vi "VendingMachine.vi"() -> ()   [LabVIEW 2022 SP3]
uses:
  <vilib>/Utility/error.llb/DialogType.ctl
  <vilib>/Instr/_visa.llb/VISA Configure Serial Port (Instr).vi
  Globalne_zmienne.vi
panel:
  out "UstalonaCena1 2":dbl=1.4256114757235e-311
  out "UstalonaCena2":dbl
  out "UstalonaCena3 2":dbl
  out "UstalonaCena4":dbl
  out "Cena 12":dbl
  out "Cena 11":dbl
  out "Cena 10":dbl
  out "Cena 9":dbl
  out "Cena 8":dbl
  out "Cena 6":dbl
  out "Cena 4":dbl
  out "Cena 5":dbl
  out "Cena 3":dbl
  out "Cena 2":dbl
  out "Cena":dbl
  out "Cena 7":dbl=1.4256114754706e-311
  in  "Ustronianka":dbl
  in  "Tarczyn":dbl
  in  "Tiger":dbl
  in  "Black":dbl
  in  "Muszynianka":dbl
  in  "Tymbark":dbl
  in  "Cappy":dbl
  in  "Nestea":dbl
  in  "Mountain Dew":dbl
  in  "Kofola":dbl
  in  "Pepsi":dbl
  in  "Coca-Cola":dbl
  out "Symulacja wydania napoju":bool
  out "Wplacone pieniadze":i32
  out "2,5":bool
  out "3":bool
  out "4,5":bool
  out "5":bool
  out "Reszta":dbl
  in  "5zl":bool
  in  "2zl":bool
  in  "1zl":bool
  out "Wybierz Numer:":i32
  in  "VISA in":refnum<visa-resource-name>
  # "Koszt wybranego napoju"
  # "Proponowane:\nUstalona cena1 = 5\nUstalona cena2 =4,5\nUstalona cena3= 3\nUstalona cena4= 2,5"
  # "Instrukcja:\n*Ustaw BoundRate na mikrokontrolerze na 228800\n\n*Ustal cene i VISA port po lewej stronie\n*Ustaw numery produktow na unikatowe dla kazdej pozycji\n\n*Za pomoca przyciskow S2 i S3 wybierz \nodpowiedni produkt\n\n*Za pomoca przyciskow wplac pieniadze\n\n*Zatwierz podwójnie przyciskajac S4"
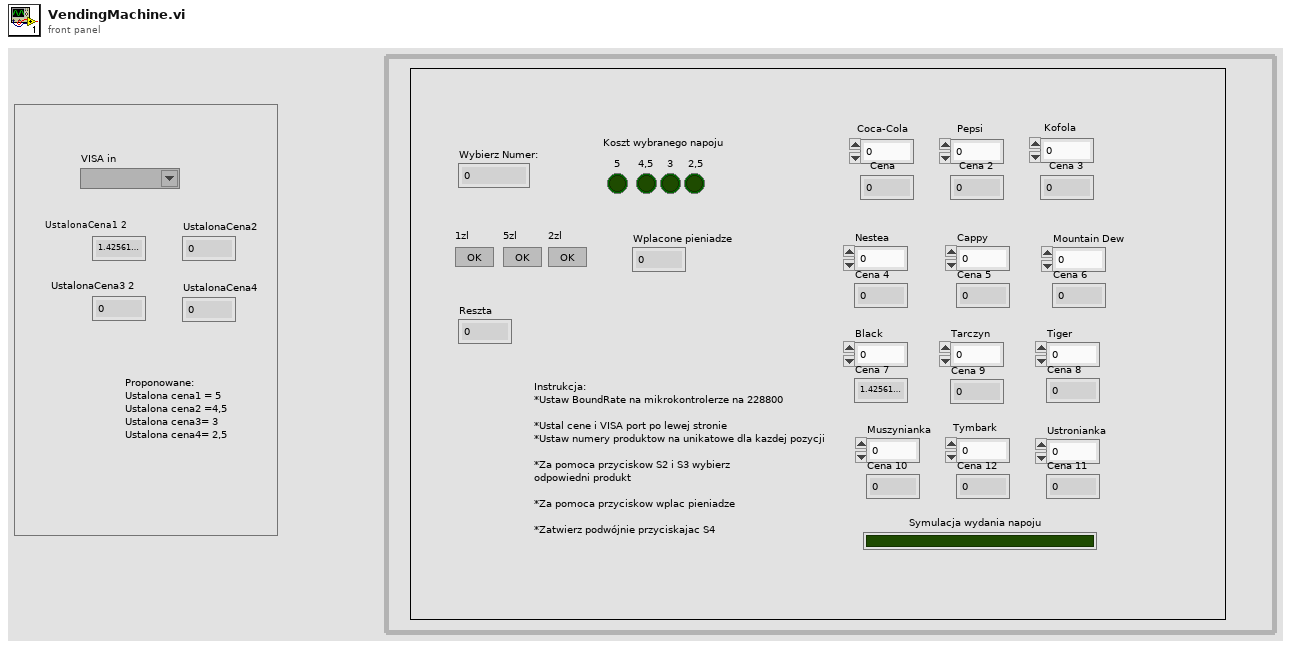
[diagram p1: front panel]
types:
  T1 = typedef "DialogType.ctl" = u16
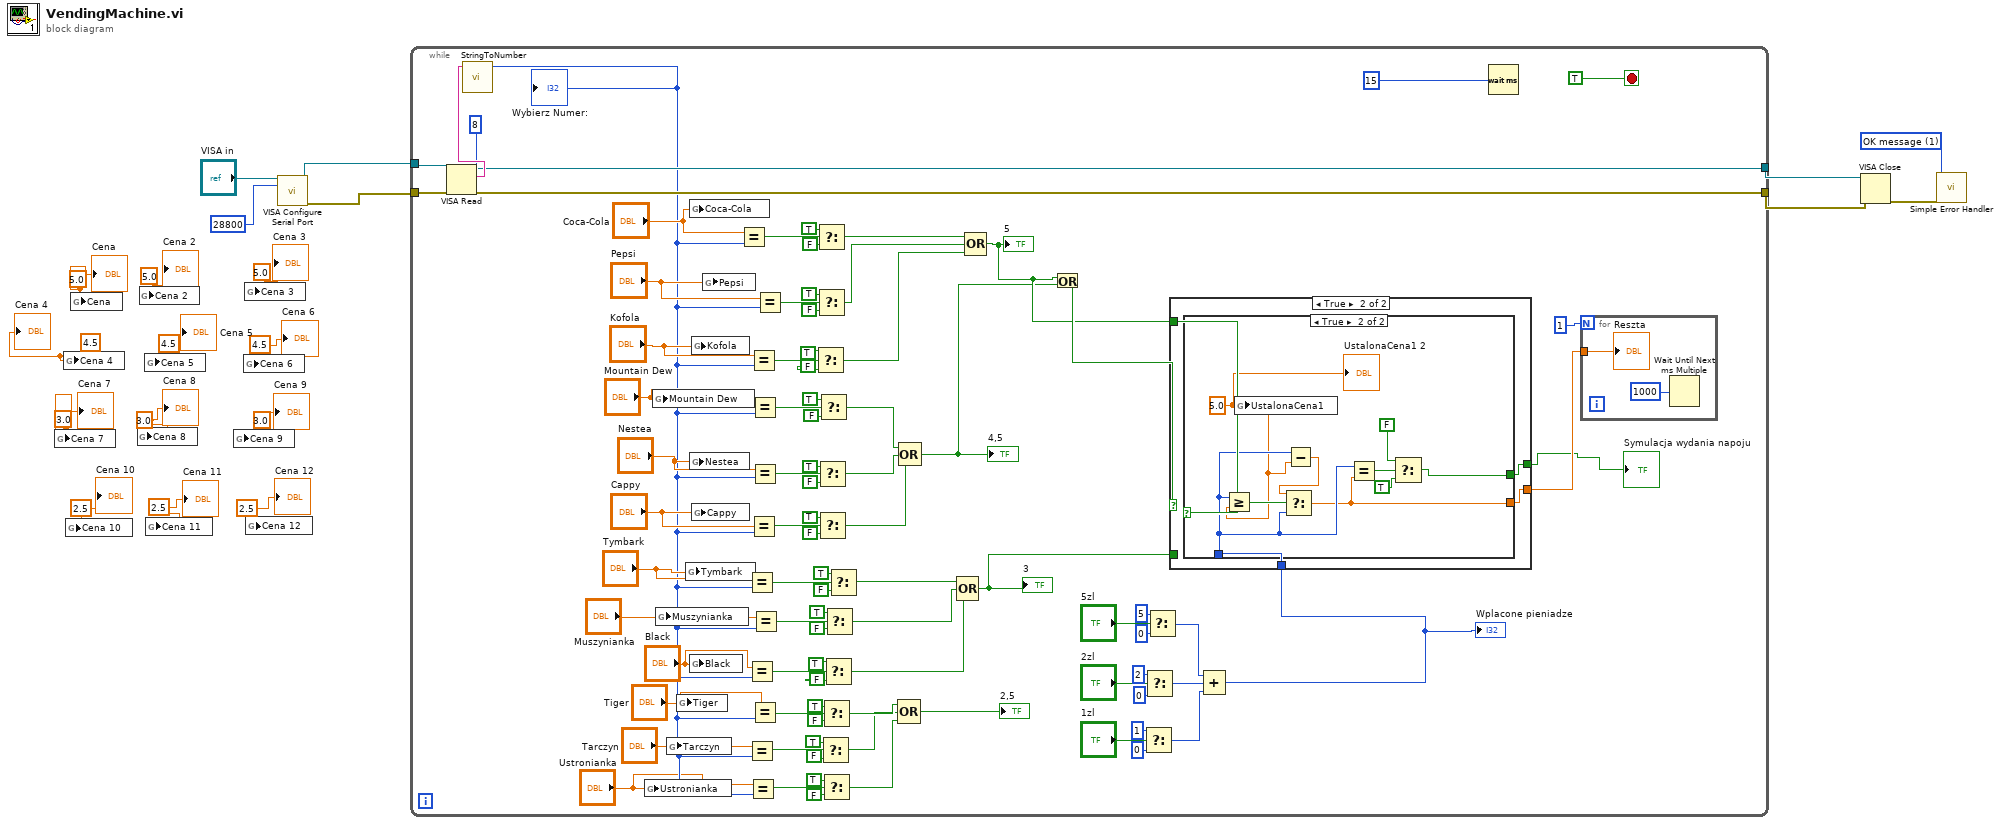
[diagram p0: block diagram]
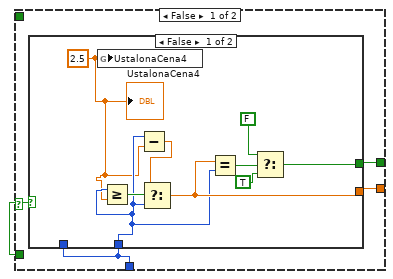
[diagram p2: hidden frame]
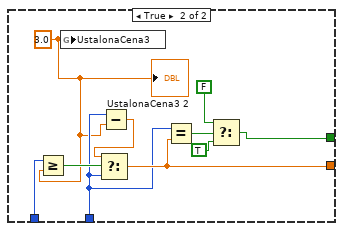
[diagram p3: hidden frame]
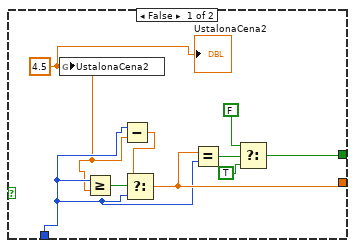
[diagram p4: hidden frame]
diagram:
  w8 = 4.5 ("Cena 5")
  w10 = 5.0 ("Cena 2")
  w7 = 4.5 ("Cena 4")
  w9 = 5.0 ("Cena 3")
  w6 = 4.5 ("Cena 6")
  w5 = 3.0 ("Cena 8")
  w3 = 2.5 ("Cena 10")
  w1 = 2.5 ("Cena 12")
  w2 = 2.5 ("Cena 11")
  w4 = 3.0 ("Cena 9")
  w12 = 3.0 ("Cena 7")
  w11 = 5.0 ("Cena")
  w16 = T1 1 items=["no dialog", "OK message", "continue or stop message", "OK message + warnings", "continue/stop + warnings"] ("type of dialog (OK msg:1)")
  n1 = global write "Globalne_zmienne.vi" "Cena 7"(w12) -> ()
  n2 = global write "Globalne_zmienne.vi" "Cena 4"(w7) -> ()
  n3 = global write "Globalne_zmienne.vi" "Cena 10"(w3) -> ()
  n4 = global write "Globalne_zmienne.vi" "Cena"(w11) -> ()
  n5 = global write "Globalne_zmienne.vi" "Cena 8"(w5) -> ()
  n6 = global write "Globalne_zmienne.vi" "Cena 2"(w10) -> ()
  n7 = global write "Globalne_zmienne.vi" "Cena 5"(w8) -> ()
  n8 = global write "Globalne_zmienne.vi" "Cena 11"(w2) -> ()
  n9 = global write "Globalne_zmienne.vi" "Cena 9"(w4) -> ()
  n10 = global write "Globalne_zmienne.vi" "Cena 6"(w6) -> ()
  n11 = global write "Globalne_zmienne.vi" "Cena 3"(w9) -> ()
  n12 = global write "Globalne_zmienne.vi" "Cena 12"(w1) -> ()
  n13 = call-poly "VISA Configure Serial Port"("VISA resource name"="VISA in", "baud rate (9600)"=u32 28800) -> ("VISA resource name out"=w18:refnum<visa-resource-name>, "error out"=w17:errorcluster)  [unwired: 12 in]
  n14 = while {
    tunnel: w18 -> [w102]
    tunnel: w17 -> [w101]
    tunnel: [w100] -> w14
    tunnel: [w99] -> w13
    stop <- TRUE stop-if-true
    n15 = VISA Read(VISA resource name=w102, byte count=u32 8, error in (no error)=w101) -> (VISA resource name out=w100:refnum<visa-resource-name>, read buffer=w110:string, error out=w99:errorcluster)  [unwired: 1 out]
    n16 = call "StringToNumber.vi"("read buffer"=w110) -> ("Numeric"=w36:i32)  [unwired: 10 in]
    "Wybierz Numer:" <- w36
    n17 = global write "Globalne_zmienne.vi" "Ustronianka"("Ustronianka") -> ()
    n18 = global write "Globalne_zmienne.vi" "Mountain Dew"("Mountain Dew") -> ()
    n19 = global write "Globalne_zmienne.vi" "Muszynianka"("Muszynianka") -> ()
    n20 = global write "Globalne_zmienne.vi" "Tarczyn"("Tarczyn") -> ()
    n21 = global write "Globalne_zmienne.vi" "Tiger"("Tiger") -> ()
    n22 = global write "Globalne_zmienne.vi" "Tymbark"("Tymbark") -> ()
    n23 = global write "Globalne_zmienne.vi" "Coca-Cola"("Coca-Cola") -> ()
    n24 = global write "Globalne_zmienne.vi" "Nestea"("Nestea") -> ()
    n25 = global write "Globalne_zmienne.vi" "Black"("Black") -> ()
    n26 = global write "Globalne_zmienne.vi" "Kofola"("Kofola") -> ()
    n27 = global write "Globalne_zmienne.vi" "Cappy"("Cappy") -> ()
    n28 = global write "Globalne_zmienne.vi" "Pepsi"("Pepsi") -> ()
    n29 = Equal?(x="Coca-Cola", y=w36) -> (x = y?=w103:bool)
    n30 = Equal?(x="Tymbark", y=w36) -> (x = y?=w79:bool)
    n31 = Equal?(x="Black", y=w36) -> (x = y?=w81:bool)
    n32 = Equal?(x="Tarczyn", y=w36) -> (x = y?=w83:bool)
    n33 = Equal?(x="Ustronianka", y=w36) -> (x = y?=w84:bool)
    n34 = Equal?(x="Kofola", y=w36) -> (x = y?=w105:bool)
    n35 = Equal?(x="Cappy", y=w36) -> (x = y?=w108:bool)
    n36 = Equal?(x="Mountain Dew", y=w36) -> (x = y?=w106:bool)
    n37 = Equal?(x="Nestea", y=w36) -> (x = y?=w107:bool)
    n38 = Equal?(x="Tiger", y=w36) -> (x = y?=w82:bool)
    n39 = Equal?(x="Muszynianka", y=w36) -> (x = y?=w80:bool)
    n40 = Equal?(x="Pepsi", y=w36) -> (x = y?=w104:bool)
    n41 = Select(t=TRUE, s=w105, f=FALSE) -> (s? t:f=w32:bool)
    n42 = Select(t=TRUE, s=w103, f=FALSE) -> (s? t:f=w34:bool)
    n43 = Select(t=TRUE, s=w104, f=FALSE) -> (s? t:f=w33:bool)
    n44 = Select(t=TRUE, s=w107, f=FALSE) -> (s? t:f=w30:bool)
    n45 = Select(t=TRUE, s=w108, f=FALSE) -> (s? t:f=w29:bool)
    n46 = Select(t=TRUE, s=w106, f=FALSE) -> (s? t:f=w31:bool)
    n47 = Select(t=TRUE, s=w83, f=FALSE) -> (s? t:f=w24:bool)
    n48 = Select(t=TRUE, s=w82, f=FALSE) -> (s? t:f=w25:bool)
    n49 = Select(t=TRUE, s=w84, f=FALSE) -> (s? t:f=w23:bool)
    n50 = Select(t=TRUE, s=w81, f=FALSE) -> (s? t:f=w26:bool)
    n51 = Select(t=TRUE, s=w80, f=FALSE) -> (s? t:f=w27:bool)
    n52 = Select(t=TRUE, s=w79, f=FALSE) -> (s? t:f=w28:bool)
    n53 = Compound Arithmetic op=OR(w25, w24, w23) -> (→"2,5":bool)
    n54 = Compound Arithmetic op=OR(w31, w30, w29) -> (w22:bool)
    "4,5" <- w22
    n55 = Compound Arithmetic op=OR(w28, w27, w26) -> (w21:bool)
    "3" <- w21
    n56 = Compound Arithmetic op=OR(w34, w33, w32) -> (w63:bool)
    "5" <- w63
    n57 = Or(x=w63, y=w22) -> (x .or. y?=w64:bool)
    n58 = Select(t=1, s="1zl", f=0) -> (s? t:f=w61:i32)
    n59 = Select(t=2, s="2zl", f=0) -> (s? t:f=w62:i32)
    n60 = Select(t=5, s="5zl", f=0) -> (s? t:f=w60:i32)
    n61 = Compound Arithmetic op=ADD(w60, w62, w61) -> (w50:i32)
    "Wplacone pieniadze" <- w50
    n62 = case shown="True" w64 {
      tunnel: w63 -> [_ w137]
      tunnel: w50 -> [w113 w136]
      tunnel: [w111 w135] -> w49
      tunnel: [w112 w134] -> w48
      tunnel: w21 -> [w114 _]
      frame False {
        n63 = case shown="False" w114 {
          tunnel: [w121 w128] -> w111
          tunnel: [w117 w127] -> w112
          tunnel: w113 -> [_ w126]
          tunnel: w113 -> [w116 w125]
          frame False {
            w115 = 2.5 ("UstalonaCena4")
            n64 = global write "Globalne_zmienne.vi" "UstalonaCena4"(w115) -> ()
            n65 = Greater Or Equal?(x=w116, y=w115) -> (x >= y?=w123:bool)
            n66 = Subtract(x=w116, y=w115) -> (x-y=w122:dbl)
            n67 = Select(t=w122, s=w123, f=w116) -> (s? t:f=w121:dbl)
            n68 = Equal?(x=w121, y=w116) -> (x = y?=w120:bool)
            n69 = Select(t=FALSE, s=w120, f=TRUE) -> (s? t:f=w117:bool)
            "UstalonaCena4" <- w115
          }
          frame True {
            w124 = 3.0 ("UstalonaCena3")
            n70 = Greater Or Equal?(x=w126, y=w124) -> (x >= y?=w133:bool)
            n71 = global write "Globalne_zmienne.vi" "UstalonaCena3"(w124) -> ()
            n72 = Subtract(x=w125, y=w124) -> (x-y=w132:dbl)
            n73 = Select(t=w132, s=w133, f=w125) -> (s? t:f=w128:dbl)
            n74 = Equal?(x=w125, y=w128) -> (x = y?=w131:bool)
            n75 = Select(t=FALSE, s=w131, f=TRUE) -> (s? t:f=w127:bool)
            "UstalonaCena3 2" <- w124
          }
        }
      }
      frame True {
        n76 = case shown="True" w137 {
          tunnel: w136 -> [w143 w150]
          tunnel: [w144 w149] -> w135
          tunnel: [w139 w148] -> w134
          frame False {
            w138 = 4.5 ("UstalonaCena2")
            n77 = global write "Globalne_zmienne.vi" "UstalonaCena2"(w138) -> ()
            n78 = Greater Or Equal?(x=w143, y=w138) -> (x >= y?=w146:bool)
            n79 = Subtract(x=w143, y=w138) -> (x-y=w145:dbl)
            n80 = Select(t=w145, s=w146, f=w143) -> (s? t:f=w144:dbl)
            n81 = Equal?(x=w144, y=w143) -> (x = y?=w142:bool)
            n82 = Select(t=FALSE, s=w142, f=TRUE) -> (s? t:f=w139:bool)
            "UstalonaCena2" <- w138
          }
          frame True {
            w147 = 5.0 ("UstalonaCena1")
            n83 = Greater Or Equal?(x=w150, y=w147) -> (x >= y?=w155:bool)
            n84 = global write "Globalne_zmienne.vi" "UstalonaCena1"(w147) -> ()
            n85 = Subtract(x=w150, y=w147) -> (x-y=w154:dbl)
            n86 = Select(t=w154, s=w155, f=w150) -> (s? t:f=w149:dbl)
            n87 = Equal?(x=w150, y=w149) -> (x = y?=w153:bool)
            n88 = Select(t=FALSE, s=w153, f=TRUE) -> (s? t:f=w148:bool)
            "UstalonaCena1 2" <- w147
          }
        }
      }
    }
    "Symulacja wydania napoju" <- w48
    n89 = Wait (ms)(milliseconds to wait=u32 15 ("General Settings:Timeout Value")) -> ()  [unwired: 1 out]
    n90 = for {
      N: 1 -> [_]
      tunnel: w49 -> [w156]
      n91 = Wait Until Next ms Multiple(millisecond multiple=u32 1000) -> ()  [unwired: 1 out]
      "Reszta" <- w156
    }
  }
  n92 = VISA Close(VISA resource name=w14, error in (no error)=w13) -> (error out=w15:errorcluster)
  n93 = call <vilib>:"Simple Error Handler.vi"("type of dialog (OK msg:1)"=w16, "error in (no error)"=w15) -> ()  [unwired: 3 in, 5 out]
  "Cena 7" <- w12
  "Cena" <- w11
  "Cena 2" <- w10
  "Cena 3" <- w9
  "Cena 5" <- w8
  "Cena 4" <- w7
  "Cena 6" <- w6
  "Cena 8" <- w5
  "Cena 9" <- w4
  "Cena 10" <- w3
  "Cena 11" <- w2
  "Cena 12" <- w1
